vi "Decision.vi"() -> ()   [LabVIEW 2010]
panel:
  out "?":string
  out "Square Root Value":dbl
  in  "Number":dbl
  in  "stop":bool
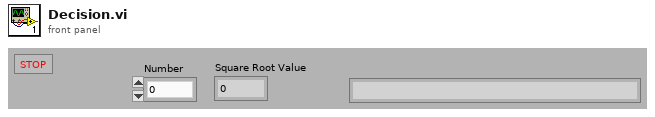
[diagram p1: front panel]
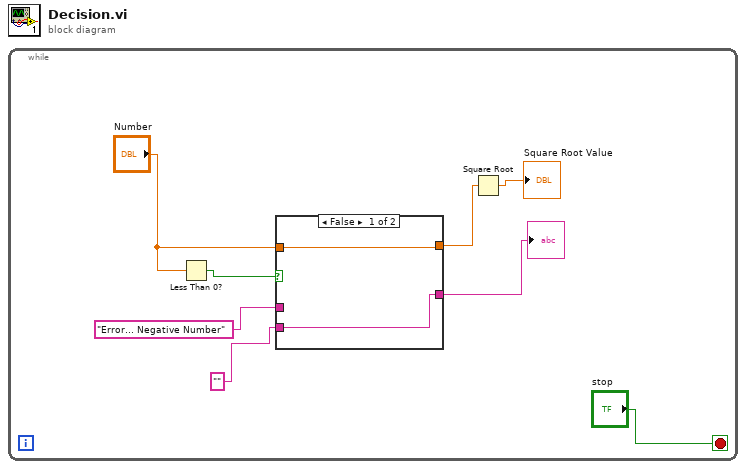
[diagram p0: block diagram]
diagram:
  n1 = while {
    stop <- "stop" stop-if-true
    n2 = Less Than 0?(x="Number") -> (x < 0?=w7:bool)
    n3 = case shown="False" w7 {
      tunnel: [w9 w12] -> w5
      tunnel: "Error... Negative Number" -> [_ w12]
      tunnel: "Number" -> [w10 w11]
      tunnel: [w10 w11] -> w3
      tunnel: "" -> [w9 _]
      frame False {
      }
      frame True {
      }
    }
    "?" <- w5
    n4 = Square Root(x=w3) -> (sqrt(x)=→"Square Root Value":dbl)
  }
